vi "Test Graph_data_collector API.vi"() -> ()   [LabVIEW 2018]
doc: "Graph_data_collector API Tester."
uses:
  Data Control.ctl
  <vilib>/Utility/error.llb/DialogType.ctl
  Graph_data_collector.lvlib
  <vilib>/measure/NI_MABase.lvlib
panel:
  in  "New_Data":bool
  out "Data 2":T1 {"tТермошкаф, °С" format="%3.1f"; "tКД30, °С" format="%3.2f"; "m весы, г" format="%.4f"; "Vо2,\nсм3" format="%.4f"; "Кпрж2 Е-3,\nмкм2" format="%.4f"; "Vо1,\nсм3" format="%.2f град.С"; "Кпрж1 Е-3,\nмкм2" format="Р2 %#.2f МПа"; "Qо1,\nсм3/мин" format="%.4f"}
  in  "frequency 2":dbl=0.001 format="%#_13g"
  in  "frequency":dbl=0.001 format="%#_13g"
  in  "Show Diagram on Init":bool
  in  "Show Block Diagram":bool
  in  "Stop Module":bool
  in  "Start Module":bool
  in  "Hide Module Panel":bool
  in  "Show Module Panel":bool
  out "Status":string
  out "Module Running?":bool
  # "This VI tests the API for the Module."
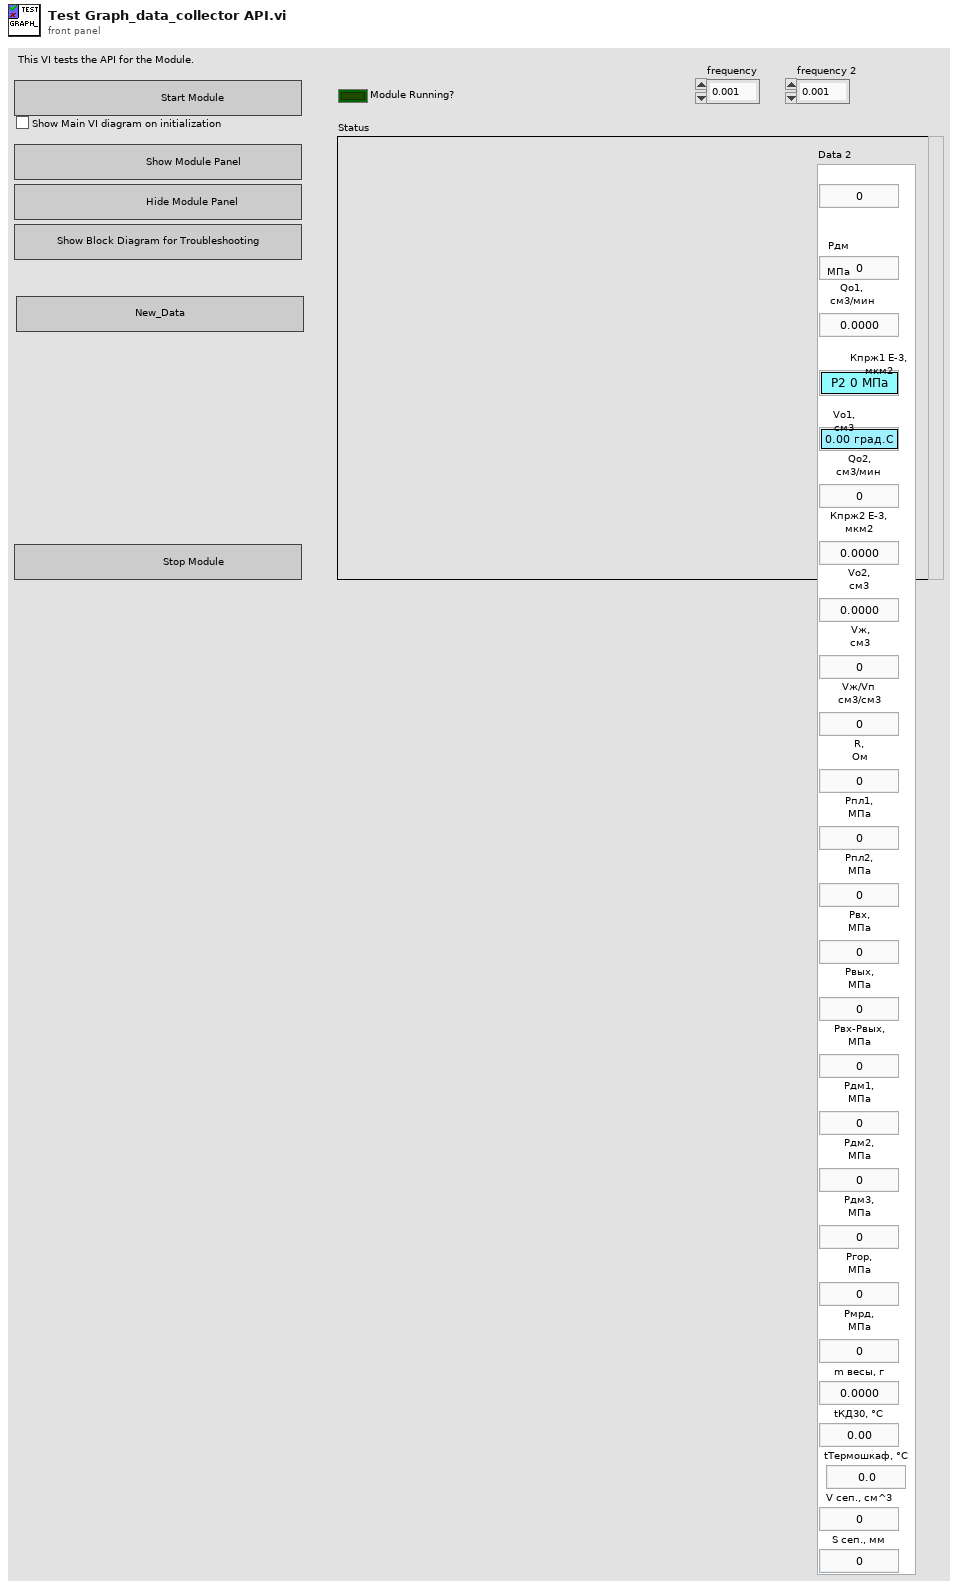
[diagram p1: front panel]
types:
  T1 = typedef "Graph_data_collector.lvlib/Data Control.ctl" = cluster{"Время":dbl, "Рдм\nрасчётное,\nМПа":dbl, "Qо1,\nсм3/мин":dbl, "Кпрж1 Е-3,\nмкм2":dbl, "Vо1,\nсм3":dbl, "Qо2,\nсм3/мин":dbl, "Кпрж2 Е-3,\nмкм2":dbl, "Vо2,\nсм3":dbl, "Vж,\nсм3":dbl, "Vж/Vп\nсм3/см3":dbl, "R,\nОм":dbl, "Рпл1,\nМПа":dbl, "Рпл2,\nМПа":dbl, "Рвх,\nМПа":dbl, "Рвых,\nМПа":dbl, "Рвх-Рвых,\nМПа":dbl, "Рдм1,\nМПа":dbl, "Рдм2,\nМПа":dbl, "Рдм3,\nМПа":dbl, "Ргор,\nМПа":dbl, "Рмрд,\nМПа":dbl, "m весы, г":dbl, "tКД30, °С ":dbl, "tТермошкаф, °С":dbl, "V сеп., см^3 ":dbl, "S сеп., мм":dbl}
  T2 = typedef "Graph_data_collector.lvlib/Broadcast Events--cluster.ctl" = cluster{"Module Did Init":refnum<user-event>, "Status Updated":refnum<user-event>, "Error Reported":refnum<user-event>, "Module Did Stop":refnum<user-event>, "Update Module Execution Status":refnum<user-event>}
  T3 = typedef "DialogType.ctl" = u16
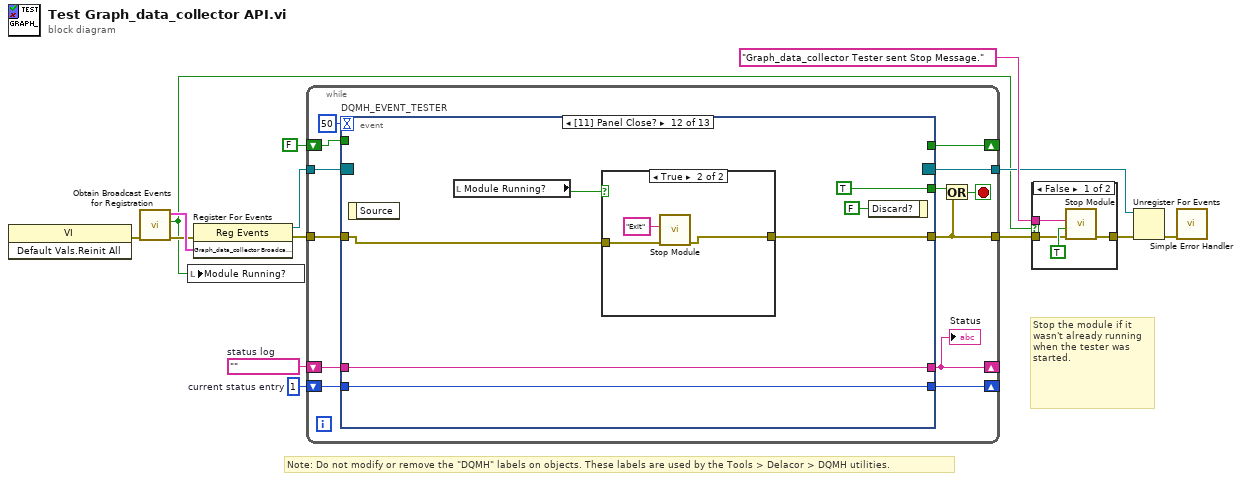
[diagram p0: block diagram]
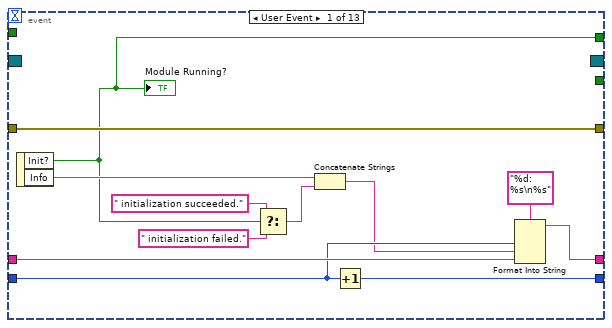
[diagram p3: hidden frame]
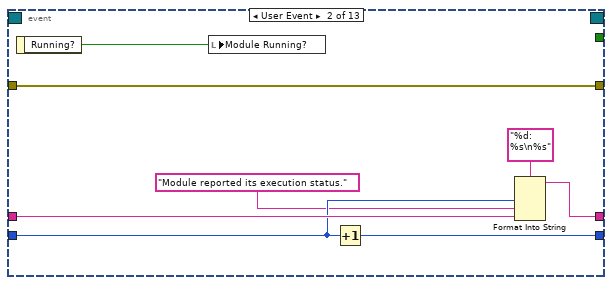
[diagram p4: hidden frame]
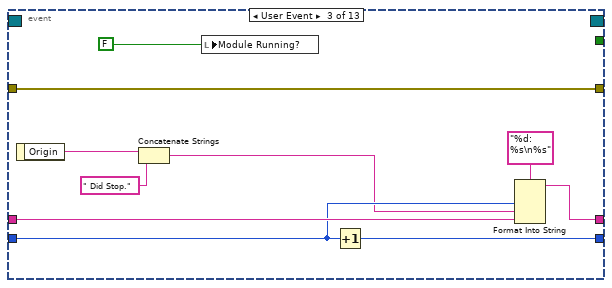
[diagram p5: hidden frame]
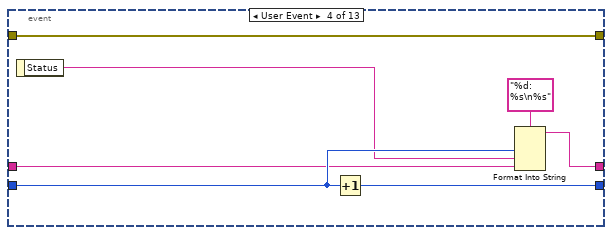
[diagram p6: hidden frame]
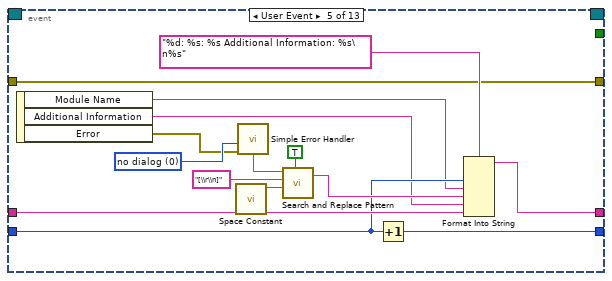
[diagram p7: hidden frame]
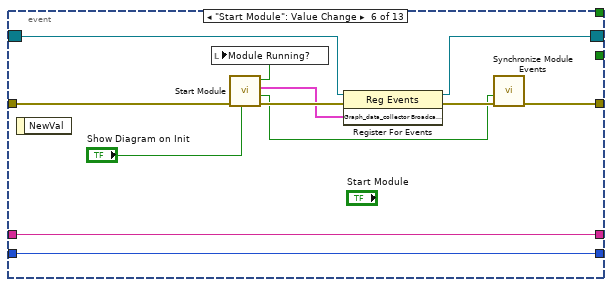
[diagram p8: hidden frame]
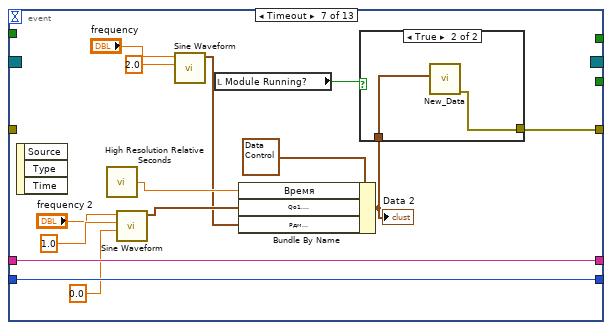
[diagram p9: hidden frame]
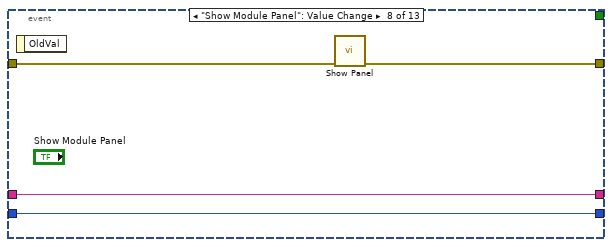
[diagram p11: hidden frame]
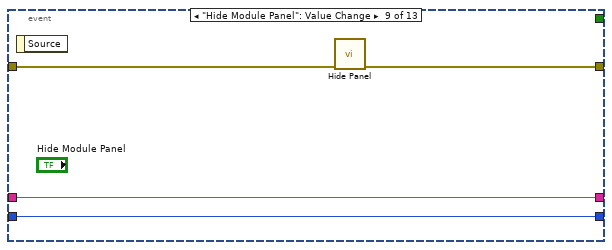
[diagram p12: hidden frame]
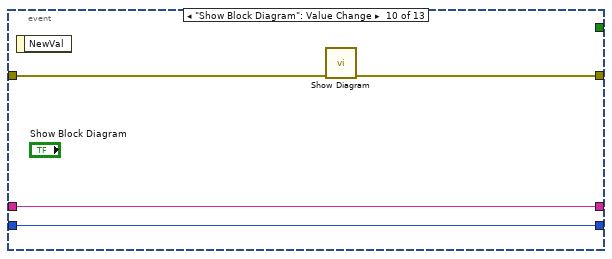
[diagram p13: hidden frame]
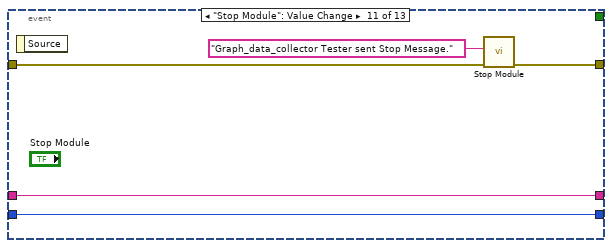
[diagram p14: hidden frame]
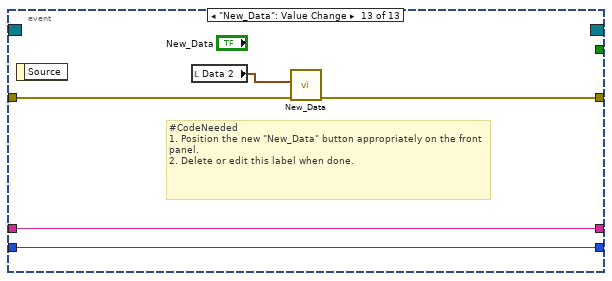
[diagram p16: hidden frame]
diagram:
  w11 = 1  # current status entry
  w12 = ""  # status log
  # "Stop the module if it wasn't already running when the tester was started."
  # "Note: Do not modify or remove the \"DQMH\" labels on objects. These labels are used by the Tools > Delacor > DQMH utilities."
  n1 = invoke class="VI" method="Default Vals.Reinit All"() -> (error out=w6:errorcluster)  [unwired: 3 in, 2 out]
  n2 = call "Obtain Broadcast Events for Registration.vi"("error in"=w6) -> ("error out"=w5:errorcluster, "Already running?"=w4:bool, "Graph_data_collector Broadcast Events"=w9:T2)  [unwired: 8 in]
  n3 = local write "Module Running?"(w4) -> ()
  n4 = register-events(error in=w5, w9) -> (reference out=w8:refnum<event-registration>, error out=w10:errorcluster)  [unwired: 1 in]
  n5 = while {
    tunnel: w8 -> [w27]
    tunnel: [w18] -> w3
    shift-right: [w22] -> _
    shift-left: w12 -> [w24]
    shift-right: [w23] -> _
    shift-left: w11 -> [w25]
    tunnel: w10 -> [w20]
    tunnel: [w19] -> w7
    shift-right: [w16] -> _
    shift-left: FALSE ("Init?") -> [w15]
    stop <- w21 stop-if-true
    n6 = event "DQMH_EVENT_TESTER" shown="[11] Panel Close?" {
      selector: w27 -> [_ _ _ _ _ w85 _ _ _ _ _ _ _]
      dyn-events: [_ _ _ _ _ w84 _ _ _ _ _ _ _] -> w19
      timeout: 50 -> [_ _ _ _ _ _ _ _ _ _ _ _ _]
      tunnel: [_ _ _ _ _ _ _ _ _ _ _ TRUE ("Discard?") _] -> w26
      tunnel: [w39 w41 w48 w58 w68 w83 w93 w111 w115 w116 w122 w125 w136] -> w18
      tunnel: w25 -> [w36 w45 w55 w61 w71 w88 w104 w109 w113 w117 w123 w129 w137]
      tunnel: w24 -> [w37 w46 w56 w60 w72 w89 w105 w110 w114 w118 w124 w130 w138]
      tunnel: [w34 w43 w53 w62 w70 w89 w105 w110 w114 w118 w124 w130 w138] -> w22
      tunnel: [w35 w44 w54 w64 w69 w88 w104 w109 w113 w117 w123 w129 w137] -> w23
      tunnel: w20 -> [w39 w41 w48 w58 w68 w82 _ w108 w112 w119 w120 w126 w139]
      tunnel: [w28 _ _ _ _ _ _ _ _ _ _ _ _] -> w16
      tunnel: w15 -> [_ _ _ _ _ _ _ _ _ _ _ _ _]
      event User Event {
        n7 = event-data() -> ("Init?"=w28:bool, "Info"=w33:string)  [unwired: 1 in]
        "Module Running?" <- w28
        n8 = Select(t=" initialization succeeded.", s=w28, f=" initialization failed.") -> (s? t:f=w29:string)
        n9 = Concatenate Strings(w33, w29) -> (w32:string)
        n10 = Increment(x=w36) -> (x+1=w35:i32)
        n11 = Format Into String(format string="%d: %s\n%s", w36, w32, w37) -> (resulting string=w34:string)  [unwired: 2 in, 1 out]
      }
      event User Event {
        n12 = event-data() -> ("Running?"=w40:bool)  [unwired: 1 in]
        n13 = local write "Module Running?"(w40) -> ()
        n14 = Increment(x=w45) -> (x+1=w44:i32)
        n15 = Format Into String(format string="%d: %s\n%s", w45, "Module reported its execution status.", w46) -> (resulting string=w43:string)  [unwired: 2 in, 1 out]
      }
      event User Event {
        n16 = event-data() -> ("Origin"=w52:string)  [unwired: 1 in]
        n17 = Concatenate Strings(w52, " Did Stop.") -> (w51:string)
        n18 = local write "Module Running?"(FALSE ("Module Did Init?")) -> ()
        n19 = Increment(x=w55) -> (x+1=w54:i32)
        n20 = Format Into String(format string="%d: %s\n%s", w55, w51, w56) -> (resulting string=w53:string)  [unwired: 2 in, 1 out]
      }
      event User Event {
        n21 = event-data() -> ("Status"=w59:string)  [unwired: 1 in]
        n22 = Increment(x=w61) -> (x+1=w64:i32)
        n23 = Format Into String(format string="%d: %s\n%s", w61, w59, w60) -> (resulting string=w62:string)  [unwired: 2 in, 1 out]
      }
      event User Event {
        w73 = T3 0 items=["no dialog", "OK message", "continue or stop message", "OK message + warnings", "continue/stop + warnings"] ("type of dialog (OK msg:1)")
        n24 = event-data() -> ("Module Name"=w67:string, "Additional Information"=w66:string, "Error"=w65:errorcluster)  [unwired: 1 in]
        n25 = call <vilib>:"Space Constant.vi"() -> ("String"=w77:string)
        n26 = call <vilib>:"Simple Error Handler.vi"("type of dialog (OK msg:1)"=w73, "error in (no error)"=w65) -> ("message"=w74:string)  [unwired: 3 in, 4 out]
        n27 = call <vilib>:"Search and Replace Pattern.vi"("string"=w74, "regular expression (\"\")"="[\\r\\n]" ("regular expression (\"\")"), "replace string (\"\")"=w77, "replace all? (F)"=TRUE ("replace all CR/LF with spaces")) -> ("result string"=w75:string)  [unwired: 1 in, 1 out]
        n28 = Increment(x=w71) -> (x+1=w69:i32)
        n29 = Format Into String(format string="%d: %s: %s Additional Information: %s\n%s", w71, w67, w75, w66, w72) -> (resulting string=w70:string)  [unwired: 2 in, 1 out]
      }
      event "Start Module": Value Change {
        n30 = event-data() -> ()  [unwired: 1 in, 1 out]
        n31 = call "Start Module.vi"("Show Main VI Diagram on Init (F)"="Show Diagram on Init", "error in"=w82) -> ("error out"=w90:errorcluster, "Wait for Event Sync?"=w87:bool, "Graph_data_collector Broadcast Events"=w86:T2, "Module Was Already Running?"=w81:bool)  [unwired: 6 in]
        n32 = local write "Module Running?"(w81) -> ()
        n33 = register-events(reference=w85, error in=w90, w86) -> (reference out=w84:refnum<event-registration>, error out=w91:errorcluster)
        n34 = call "Synchronize Module Events.vi"("error in"=w91, "Wait for Event Sync?"=w87) -> ("error out"=w83:errorcluster)  [unwired: 9 in]
      }
      event Timeout {
        n35 = event-data() -> ()  [unwired: 1 in, 3 out]
        n36 = call <vilib>:"High Resolution Relative Seconds.vi"() -> ("relative seconds"=w102:dbl)
        n37 = call <vilib>:"Sine Waveform.vi"("phase"=0.0, "amplitude"=1.0, "frequency"="frequency 2") -> ("signal out"=w101:waveform(dbl))  [unwired: 7 in, 1 out]
        n38 = call <vilib>:"Sine Waveform.vi"("amplitude"=2.0, "frequency"="frequency") -> ("signal out"=w95:waveform(dbl))  [unwired: 8 in, 1 out]
        n39 = local read "Module Running?"() -> (w92:bool)
        n40 = Bundle By Name(cluster=T1 {"Время"=0.0, "Рдм\nрасчётное,\nМПа"=0.0, "Qо1,\nсм3/мин"=0.0, "Кпрж1 Е-3,\nмкм2"=0.0, "Vо1,\nсм3"=0.0, "Qо2,\nсм3/мин"=0.0, "Кпрж2 Е-3,\nмкм2"=0.0, "Vо2,\nсм3"=0.0, "Vж,\nсм3"=0.0, "Vж/Vп\nсм3/см3"=0.0, "R,\nОм"=0.0, "Рпл1,\nМПа"=0.0, "Рпл2,\nМПа"=0.0, "Рвх,\nМПа"=0.0, "Рвых,\nМПа"=0.0, "Рвх-Рвых,\nМПа"=0.0, "Рдм1,\nМПа"=0.0, "Рдм2,\nМПа"=0.0, "Рдм3,\nМПа"=0.0, "Ргор,\nМПа"=0.0, "Рмрд,\nМПа"=0.0, "m весы, г"=0.0, "tКД30, °С "=0.0, "tТермошкаф, °С"=0.0, "V сеп., см^3 "=0.0, "S сеп., мм"=0.0} ("Data 2"), "Время"=w102, "Qо1,\nсм3/мин"=w101, "Рдм\nрасчётное,\nМПа"=w95) -> (w94:T1)
        "Data 2" <- w94
        n41 = case shown="True" w92 {
          tunnel: w94 -> [_ w107]
          tunnel: [_ w106] -> w93
          frame False {
          }
          frame True {
            n42 = call "New_Data.vi"("Graph_Data"=w107) -> ("error out"=w106:errorcluster)  [unwired: 10 in]
          }
        }
      }
      event "Show Module Panel": Value Change {
        n43 = event-data() -> ()  [unwired: 1 in, 1 out]
        n44 = call "Show Panel.vi"("error in (no error)"=w108) -> ("error out"=w111:errorcluster)  [unwired: 10 in]
      }
      event "Hide Module Panel": Value Change {
        n45 = event-data() -> ()  [unwired: 1 in, 1 out]
        n46 = call "Hide Panel.vi"("error in (no error)"=w112) -> ("error out"=w115:errorcluster)  [unwired: 10 in]
      }
      event "Show Block Diagram": Value Change {
        n47 = event-data() -> ()  [unwired: 1 in, 1 out]
        n48 = call "Show Diagram.vi"("error in (no error)"=w119) -> ("error out"=w116:errorcluster)  [unwired: 10 in]
      }
      event "Stop Module": Value Change {
        n49 = event-data() -> ()  [unwired: 1 in, 1 out]
        n50 = call "Stop Module.vi"("error in"=w120, "Origin"="Graph_data_collector Tester sent Stop Message.") -> ("error out"=w122:errorcluster)  [unwired: 9 in]
      }
      event Panel Close? {
        n51 = event-data() -> ()  [unwired: 1 in, 1 out]
        n52 = local read "Module Running?"() -> (w127:bool)
        n53 = case shown="True" w127 {
          tunnel: w126 -> [_ w134]
          tunnel: [_ w133] -> w125
          frame False {
          }
          frame True {
            n54 = call "Stop Module.vi"("error in"=w134, "Origin"="Exit") -> ("error out"=w133:errorcluster)  [unwired: 9 in]
          }
        }
        n55 = event-data("Discard?"=FALSE) -> ()  [unwired: 1 in, 1 out]
      }
      event "New_Data": Value Change {
        # "#CodeNeeded\n1. Position the new \"New_Data\" button appropriately on the front panel.\n2. Delete or edit this label when done."
        n56 = event-data() -> ()  [unwired: 1 in, 1 out]
        n57 = local read "Data 2"() -> (w135:T1)
        n58 = call "New_Data.vi"("error in"=w139, "Graph_Data"=w135) -> ("error out"=w136:errorcluster)  [unwired: 9 in]
      }
    }
    "Status" <- w22
    n59 = Or(x=w26, y=w18) -> (x .or. y?=w21:bool)
  }
  n60 = case shown="False" w4 {
    tunnel: [w143 w144] -> w14
    tunnel: "Graph_data_collector Tester sent Stop Message." ("Origin") -> [w142 _]
    tunnel: w3 -> [w140 w144]
    frame False {
      n61 = call "Stop Module.vi"("error in"=w140, "Wait for Module to Stop? (F)"=TRUE ("Wait for Module to stop?"), "Origin"=w142) -> ("error out"=w143:errorcluster)  [unwired: 8 in]
    }
    frame True {
    }
  }
  n62 = Unregister For Events(event registration refnum=w7, error in=w14) -> (error out=w2:errorcluster)
  n63 = call <vilib>:"Simple Error Handler.vi"("error in (no error)"=w2) -> ()  [unwired: 4 in, 5 out]
